vi "Source_ROI Values format specifier-norm values precision.vi"() -> (3 "format (%.3f)":string)   [LabVIEW 2013]
panel:
  # "SUBROUTINE"
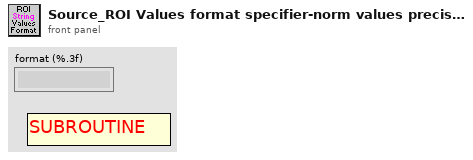
[diagram p1: front panel]
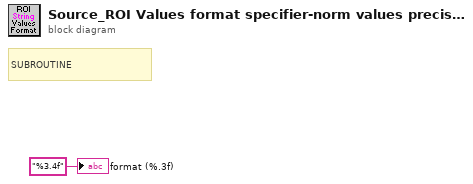
[diagram p0: block diagram]
diagram:
  # "SUBROUTINE"
  "format (%.3f)" <- "%3.4f" ("format (%.3f)")
